vi "test_SessionsRegistered_ReserveSessions_IndicatesSessionsExist.vi"(8 "error in":errorcluster) -> (0 "error out":errorcluster, 2 "result":string, 3 "pass":bool)   [LabVIEW 2020, in "MeasurementServerTests.lvlib" / "Session Reservation Tests.lvlib"]
uses:
  Session Reservation Tests.lvlib
  Runtime/MeasurementLink Session Management Client/RPC Messages/ni_measurementlink_PinMapContext.ctl
  Runtime/MeasurementLink Session Management/Session Reservation/Session Reservation.lvclass/Session Reservation.ctl
  Runtime/MeasurementLink Session Management/Session Reservation/Merge Invalid DVR Error.vi
  Helpers/Pin Map XML Strings Global.vi
  Runtime/MeasurementLink Session Management/Session Reservation/Is DVR Valid.vi
  Runtime/MeasurementLink Measurement Server/Helpers/Error Strings Global Internal.vi
  <vilib>/Utility/error.llb/Error Cluster From Error Code.vi
  MeasurementServerTests.lvlib
  Runtime/MeasurementLink Session Management/Session Reservation/Session Reservation.lvclass
  Runtime/MeasurementLink Session Management Client/MeasurementLink Session Management Client.lvlib
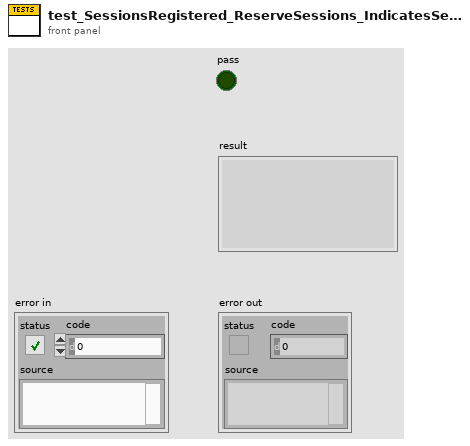
[diagram p1: front panel]
types:
  T1 = typedef "MeasurementLink Session Management Client.lvlib/ni_measurementlink_PinMapContext.ctl" = cluster{"pin_map_id":string, "sites":i32[]}
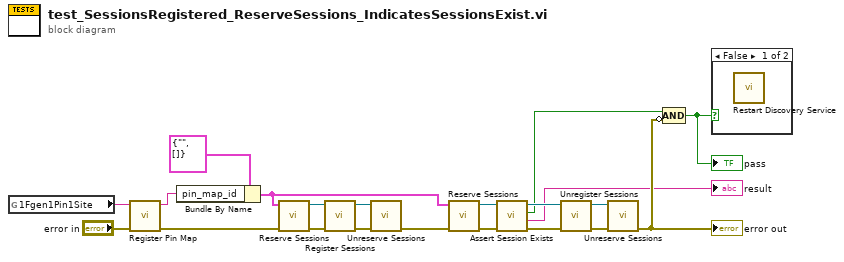
[diagram p0: block diagram]
diagram:
  n1 = global read "Pin Map XML Strings Global.vi" "1Fgen1Pin1Site"() -> (w18:string)
  n2 = call "Register Pin Map.vi"("error in"="error in", "pin map xml"=w18) -> ("error out"=w21:errorcluster, "pin map id"=w19:string)  [unwired: 8 in]
  n3 = Bundle By Name(cluster=T1 {"pin_map_id"="", "sites"=[]} ("pin map context"), "pin_map_id"=w19) -> (w16:T1)
  n4 = call "Reserve Sessions.vi"("error in"=w21, "pin map context"=w16) -> ("error out"=w15:errorcluster, "session reservation out"=w13:refnum<class "Session Reservation.lvclass">)  [unwired: 8 in]
  n5 = call "Register Sessions.vi"("error in"=w15, "session reservation in"=w13) -> ("error out"=w14:errorcluster, "session reservation out"=w12:refnum<class "Session Reservation.lvclass">)  [unwired: 8 in]
  n6 = call "Unreserve Sessions.vi"("error in"=w14, "session reservation in"=w12) -> ("error out"=w11:errorcluster)  [unwired: 9 in]
  n7 = call "Reserve Sessions.vi"("error in"=w11, "pin map context"=w16) -> ("error out"=w6:errorcluster, "session reservation out"=w4:refnum<class "Session Reservation.lvclass">)  [unwired: 8 in]
  n8 = call "Assert Session Exists.vi"("error in"=w6, "session reservation in"=w4) -> ("error out"=w5:errorcluster, "result"=→"result":string, "pass"=w2:bool, "session reservation out"=w3:refnum<class "Session Reservation.lvclass">)  [unwired: 6 in]
  n9 = call "Unregister Sessions.vi"("error in"=w5, "session reservation in"=w3) -> ("error out"=w8:errorcluster, "session reservation out"=w7:refnum<class "Session Reservation.lvclass">)  [unwired: 8 in]
  n10 = call "Unreserve Sessions.vi"("error in"=w8, "session reservation in"=w7) -> ("error out"=w10:errorcluster)  [unwired: 9 in]
  "error out" <- w10
  n11 = Compound Arithmetic op=AND(w2, invert w10) -> (w9:bool)
  "pass" <- w9
  n12 = case shown="False" w9 {
    frame False {
      n13 = call "Restart Discovery Service.vi"() -> ()  [unwired: 11 in, 1 out]
    }
    frame True {
    }
  }
